vi "Linspace.vi"(1 "Stop_value":dbl, 2 "Start_value":dbl, 3 "Num":i32) -> (0 "Output_array":dbl[](array[numeric]))   [LabVIEW 2020]
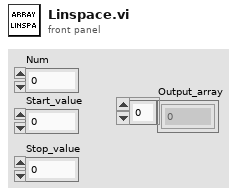
[diagram p1: front panel]
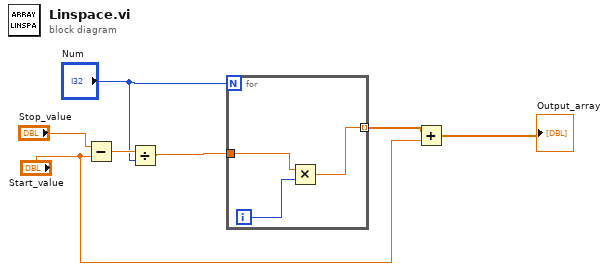
[diagram p0: block diagram]
diagram:
  n1 = Subtract(x="Stop_value", y="Start_value") -> (x-y=w6:dbl)
  n2 = Divide(x=w6, y="Num") -> (x/y=w4:dbl)
  n3 = for {
    N: "Num" -> [_]
    tunnel: w4 -> [w9]
    tunnel: [w8] -> w3 mode=indexing
    i -> [w10]
    n4 = Multiply(x=w9, y=w10) -> (x*y=w8:dbl)
  }
  n5 = Add(x=w3, y="Start_value") -> (x+y=→"Output_array":dbl[])
